vi "WriteFile.vi"(0 "File Path":path, 1 "Initialize Settings":T1, 2 "Channel(s) Settings":T4 {"Channel(s)"."Verticle Settings"."Vertical Coupling" items=["AC", "DC", "Ground"]; "Channel(s)"."Verticle Settings"."Probe Attenuation" format="%.1f"; "Channel(s)"."Verticle Settings"."Vertical Offset" format="%.2p"; "Channel(s)"."Verticle Settings"."Vertical Range" format="%.2f"; "Channel(s)"."Maximum Input Frequency" format="%.2f"}, 3 "Horizontal Settings":T2={"Continuous"=FALSE, "EnableAveraging"=FALSE, "Number Averages"=0, "Measurement Timeout"=0.0, "Min Record Length"=1000, "Min Sample Rate"=10000000.0, "Enforce Realtime"=TRUE, "Sampling Mode "=enum."Real Time", "Interpolation"=enum."No Interpolation", "Type"=enum."Normal", "StartTime"=0.0, "Time Per Record"=0.0, "Number of Points Minimum"=0} {"Min Sample Rate" step=1000000.0 format="%#.2p"}, 4 "Specific&CommonTriggerProperties":T3={"Common Trigger Settings"={"Trigger Delay"=0.0, "Reference Position"=50.0, "Trigger Modifier"=2, "Auto Triggered"=FALSE}, "Specific Trigger Settings"={"Source"="", "Holdoff"=0.0, "Level"=0.0, "Trigger Slope"=enum."Negative", "Type"=enum."Immediate", "Window Mode"=0, "Low Level"=-0.1, "High Level"=0.1, "Coupling"=1, "Hysteresis"=0.05}} {"Specific Trigger Settings"."Hysteresis" format="%.2f"; "Specific Trigger Settings"."Coupling" items=["AC"=0, "DC"=1, "HF Reject"=3, "LF Reject"=4, "AC Plus HF Reject"=1001]; "Specific Trigger Settings"."High Level" format="%.2f"; "Specific Trigger Settings"."Low Level" format="%.2f"; "Specific Trigger Settings"."Window Mode" items=["Entering", "Leaving"]; "Common Trigger Settings"."Trigger Modifier" items=["None"=1, "Auto Trigger"=2]; "Common Trigger Settings"."Reference Position" format="%.1f"; "Common Trigger Settings"."Trigger Delay" format="%#.4p"}, 5 "Error In":errorcluster) -> (19 "error out":errorcluster)   [LabVIEW 2018, in "ScopePlugins.lvlib" / "ScopePluginsBase.lvclass"]
uses:
  ScopePluginsBase.lvclass
  Typedefs/ChannelSetting(s).ctl
  Typedefs/TriggerSettings.ctl
  Typedefs/HorizontalSettings.ctl
  Typedefs/InitializationSettings.ctl
  <vilib>/Utility/config.llb/NI_LVConfig.lvlib
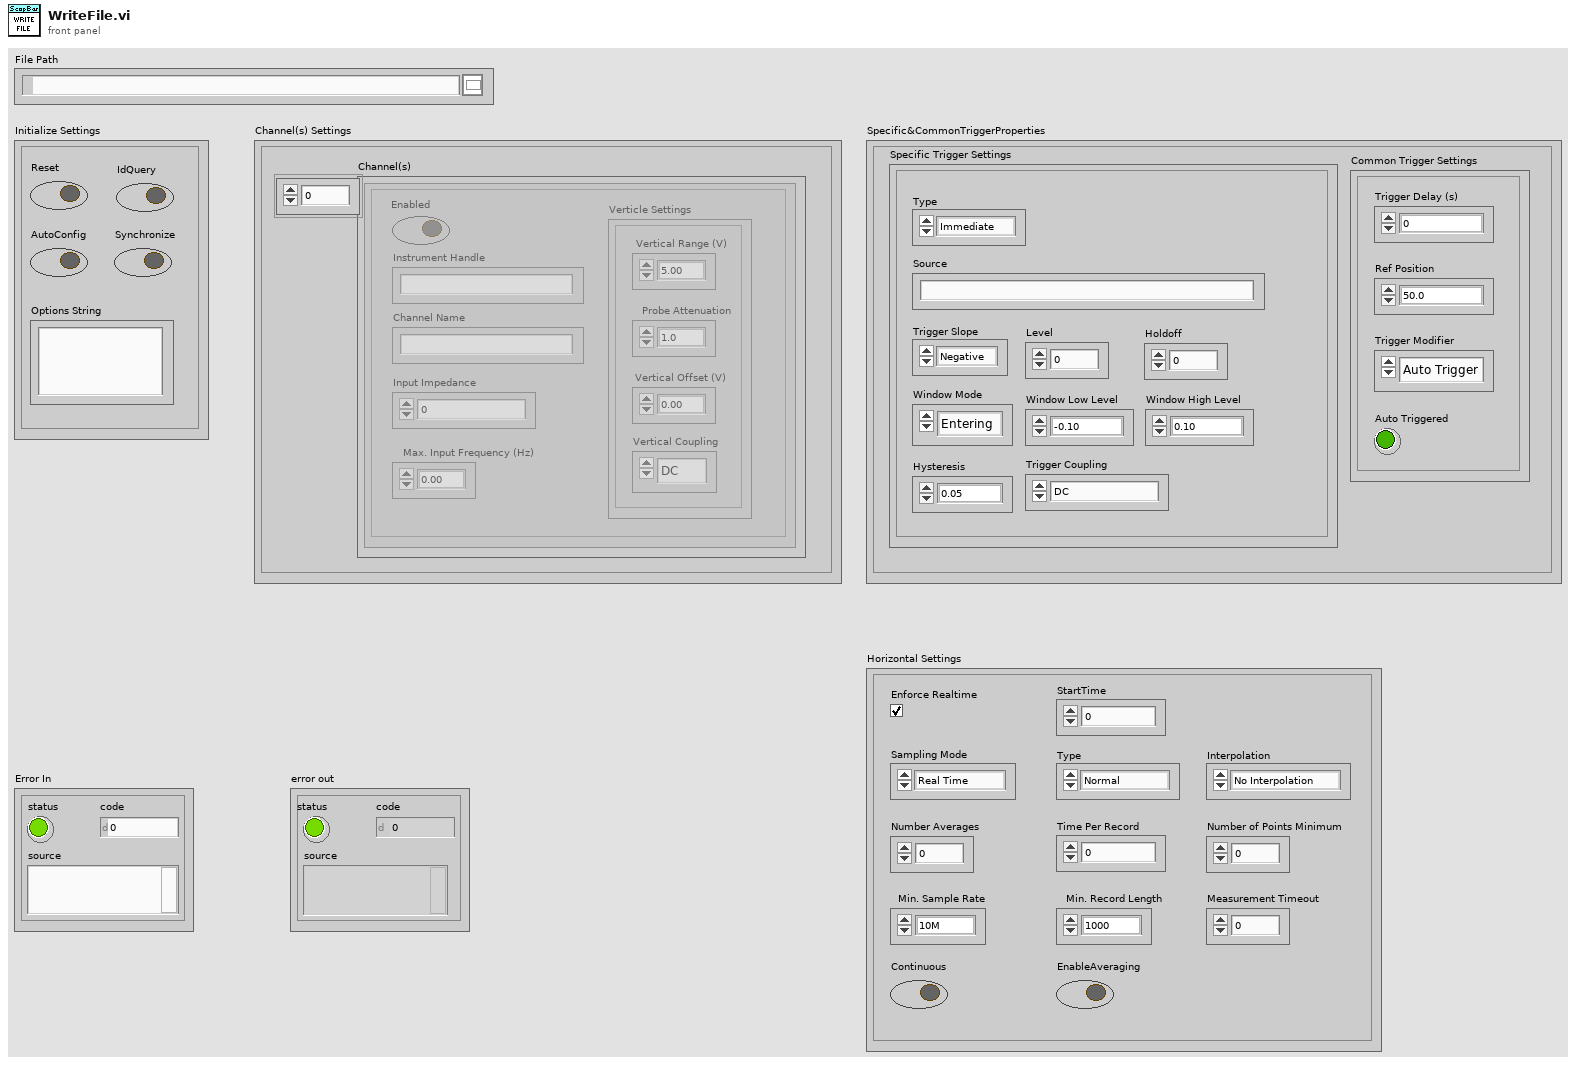
[diagram p1: front panel]
types:
  T1 = typedef "ScopePlugins.lvlib/ScopePluginsBase.lvclass/InitializationSettings.ctl" = cluster{"Reset":bool, "IdQuery":bool, "AutoConfig":bool, "Options String":string, "Synchronize":bool}
  T2 = typedef "ScopePlugins.lvlib/ScopePluginsBase.lvclass/HorizontalSettings.ctl" = cluster{"Continuous":bool, "EnableAveraging":bool, "Number Averages":i32, "Measurement Timeout":dbl, "Min Record Length":i32, "Min Sample Rate":dbl, "Enforce Realtime":bool, "Sampling Mode ":enum16{"Real Time", "Equivalent Time", "Segment", "Real Time Peak Detect", "Real Time High Resolution", "Peak Detect Segment", "High Resolution Segment"}, "Interpolation":enum16{"No Interpolation", "sin(x)/x", "linear", "1 Point sin(x)/x", "2 Point sin(x)/x", "4 Point sin(x)/x", "8 Point sin(x)/x", "16 Point sin(x)/x"}, "Type":enum16{"Normal", "PeakDetect", "HighRes", "Envelope", "Average"}, "StartTime":dbl, "Time Per Record":dbl, "Number of Points Minimum":i32}
  T3 = typedef "ScopePlugins.lvlib/ScopePluginsBase.lvclass/TriggerSettings.ctl" = cluster{"Common Trigger Settings":cluster{"Trigger Delay":dbl, "Reference Position":dbl, "Trigger Modifier":i32, "Auto Triggered":bool}, "Specific Trigger Settings":cluster{"Source":string, "Holdoff":dbl, "Level":dbl, "Trigger Slope":enum16{"Negative", "Positive"}, "Type":enum16{"Immediate", "Edge", "Digitial", "Window", "Hysteresis", "Width", "Runt", "Glitch", "TV", "AC Line"}, "Window Mode":i32, "Low Level":dbl, "High Level":dbl, "Coupling":u16, "Hysteresis":dbl}}
  T4 = typedef "ScopePlugins.lvlib/ScopePluginsBase.lvclass/ChannelSetting(s).ctl" = cluster{"Number of Channels":i32, "Channel(s)":cluster{"Enabled":bool, "Instrument Handle":string, "Channel Name":string, "Maximum Input Frequency":dbl, "Verticle Settings":cluster{"Vertical Range":dbl, "Vertical Offset":dbl, "Probe Attenuation":dbl, "Vertical Coupling":i32}, "Connected":bool, "Input Impedance":dbl}[]}
  T5 = typedef "NI_LVConfig.lvlib/Config Data RefNum.ctl" = refnum<k1>
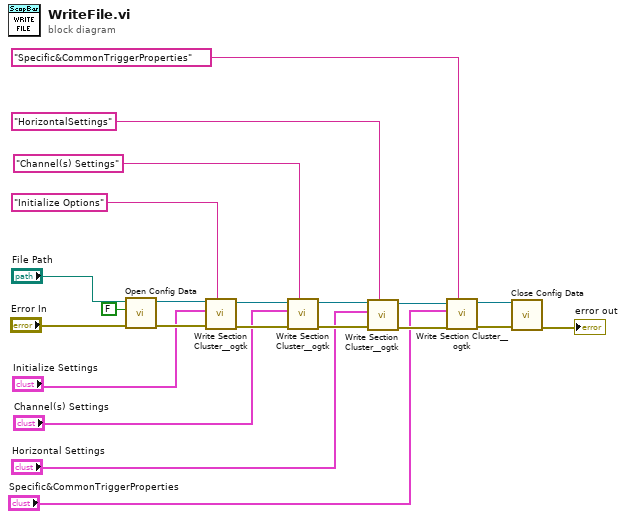
[diagram p0: block diagram]
diagram:
  n1 = call <vilib>:"Open Config Data.vi"("error in (no error)"="Error In", "create file if necessary (T)"=FALSE, "configuration file path"="File Path") -> ("error out"=w21:errorcluster, "refnum"=w22:T5)  [unwired: 6 in, 1 out]
  n2 = call <userlib>:"Write Section Cluster__ogtk.vi"("section (optional)"="Initialize Options", "error in (no error)"=w21, "Section Formatted Cluster"="Initialize Settings", "refnum"=w22) -> ("error out"=w20:errorcluster, "dup refnum"=w18:T5)  [unwired: 6 in]
  n3 = call <userlib>:"Write Section Cluster__ogtk.vi"("section (optional)"="Channel(s) Settings", "error in (no error)"=w20, "Section Formatted Cluster"="Channel(s) Settings", "refnum"=w18) -> ("error out"=w19:errorcluster, "dup refnum"=w17:T5)  [unwired: 6 in]
  n4 = call <userlib>:"Write Section Cluster__ogtk.vi"("section (optional)"="HorizontalSettings", "error in (no error)"=w19, "Section Formatted Cluster"="Horizontal Settings", "refnum"=w17) -> ("error out"=w16:errorcluster, "dup refnum"=w15:T5)  [unwired: 6 in]
  n5 = call <userlib>:"Write Section Cluster__ogtk.vi"("section (optional)"="Specific&CommonTriggerProperties", "error in (no error)"=w16, "Section Formatted Cluster"="Specific&CommonTriggerProperties", "refnum"=w15) -> ("error out"=w14:errorcluster, "dup refnum"=w13:T5)  [unwired: 6 in]
  n6 = call <vilib>:"Close Config Data.vi"("error in (no error)"=w14, "refnum"=w13) -> ("error out"=→"error out":errorcluster)  [unwired: 8 in, 1 out]
